vi "Create Folder.vi"(8 "error in (no error)":errorcluster, 11 "File or Folder":path) -> (0 "error out":errorcluster, 1 "Created Folder":bool, 2 "Folder Path":path, 3 "dup File":path)   [LabVIEW 2018]
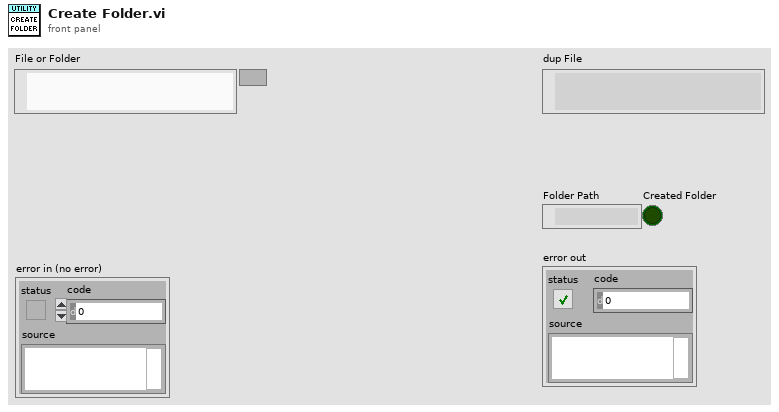
[diagram p1: front panel]
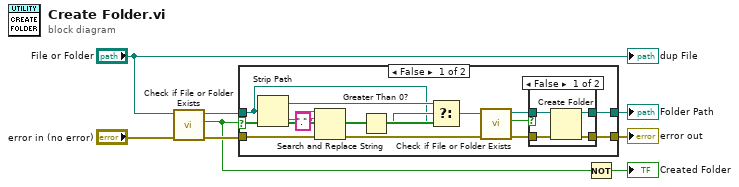
[diagram p0: block diagram]
diagram:
  n1 = call <vilib>:"Check if File or Folder Exists.vi"("error in (no error)"="error in (no error)", "path"="File or Folder") -> ("error out"=w3:errorcluster, "file or folder exists?"=w2:bool, "dup path"=w1:path)  [unwired: 7 in]
  n2 = case shown="False" w2 {
    tunnel: w1 -> [w14 w30]
    tunnel: w3 -> [w20 w29]
    tunnel: [w22 w29] -> w8
    tunnel: [w21 w30] -> w7
    frame False {
      n3 = Strip Path(path=w14) -> (stripped path=w15:path, name=w19:string)
      n4 = Search and Replace String(input string=w19, search string=".", error in=w20) -> (number of replacements=w17:i32, error out=w12:errorcluster)  [unwired: 5 in, 2 out]
      n5 = Greater Than 0?(x=w17) -> (x > 0?=w16:bool)
      n6 = Select(t=w15, s=w16, f=w14) -> (s? t:f=w13:path)
      n7 = call <vilib>:"Check if File or Folder Exists.vi"("error in (no error)"=w12, "path"=w13) -> ("error out"=w11:errorcluster, "file or folder exists?"=w10:bool, "dup path"=w9:path)  [unwired: 7 in]
      n8 = case shown="False" w10 {
        tunnel: [w26 w27] -> w22
        tunnel: [w25 w28] -> w21
        tunnel: w11 -> [w24 w27]
        tunnel: w9 -> [w23 w28]
        frame False {
          n9 = Create Folder(path (use dialog)=w23, error in=w24) -> (created path=w25:path, error out=w26:errorcluster)  [unwired: 1 in, 1 out]
        }
        frame True {
        }
      }
    }
    frame True {
    }
  }
  "error out" <- w8
  "Folder Path" <- w7
  n10 = Not(x=w2) -> (.not. x?=→"Created Folder":bool)
  "dup File" <- "File or Folder"
